vi "Countdown (SubVI).vi"(9 "s":bool) -> (0 "x/y":dbl format="%<%M:%S>t")   [LabVIEW 2020]
panel:
  out "8bit integer 2":i8 format="%08b"
  out "-1, 0, 1":dbl
  out "8bit integer":i8 format="%08b"
  in  "stop":bool
  # "T"
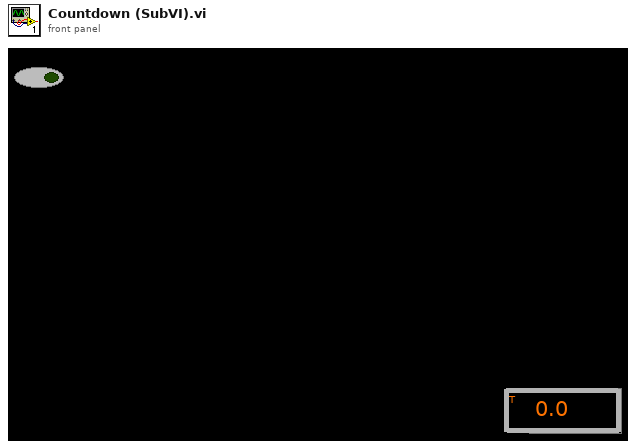
[diagram p1: front panel]
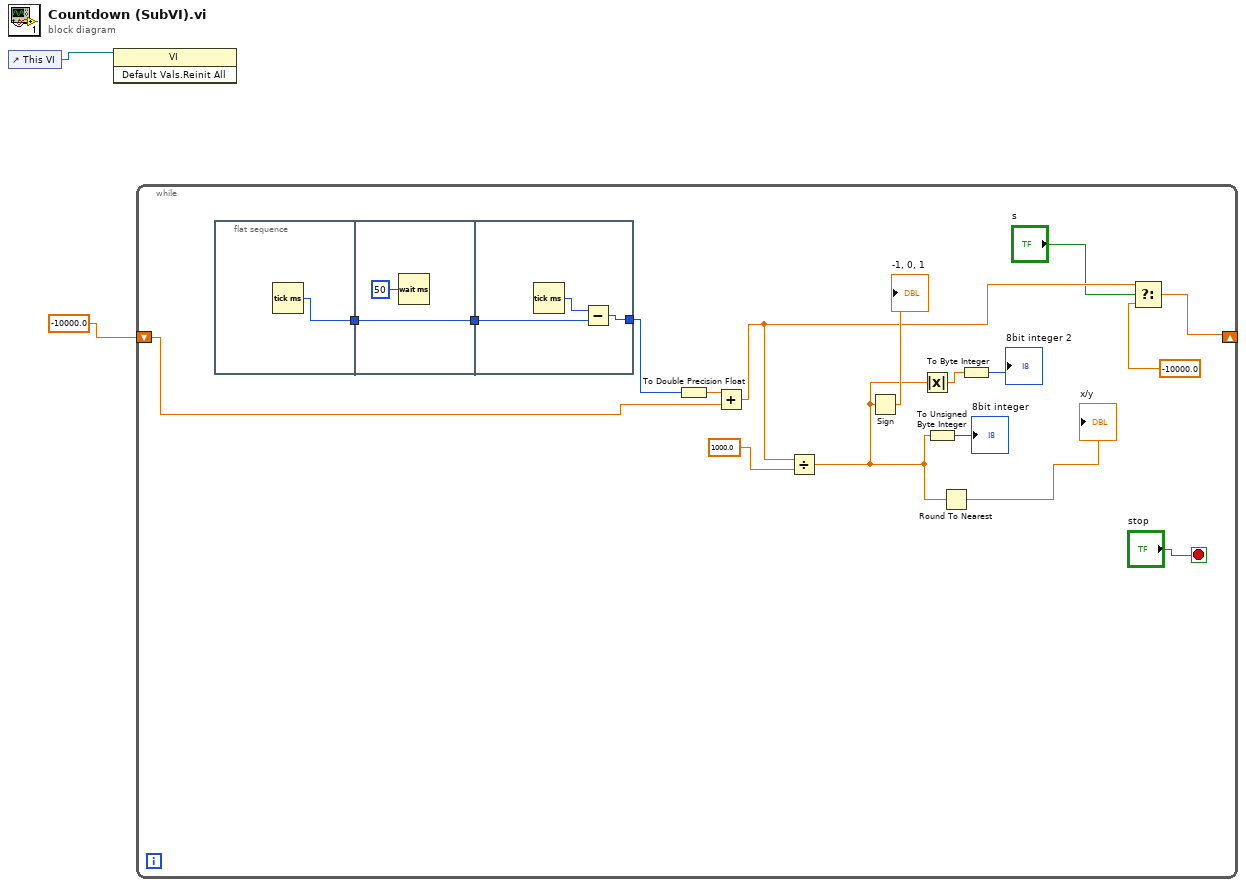
[diagram p0: block diagram]
diagram:
  n1 = control-ref of="This VI"() -> (w2:refnum<vi>)
  n2 = invoke class="VI" method="Default Vals.Reinit All"(reference=w2) -> ()  [unwired: 2 in, 3 out]
  n3 = while {
    shift-right: [w7] -> _
    shift-left: -10000.0 -> [w18]
    stop <- "stop" stop-if-true
    n4 = flat-sequence {
      tunnel: [w20] -> w16
      tunnel: w16 -> [w22]
      tunnel: [w22] -> w15
      tunnel: w15 -> [w24]
      tunnel: [w23] -> w14
      frame #0 {
        n5 = Tick Count (ms)() -> (millisecond timer value=w20:u32)
      }
      frame #1 {
        n6 = Wait (ms)(milliseconds to wait=u32 50) -> ()  [unwired: 1 out]
      }
      frame #2 {
        n7 = Tick Count (ms)() -> (millisecond timer value=w25:u32)
        n8 = Subtract(x=w25, y=w24) -> (x-y=w23:u32)
      }
    }
    n9 = To Double Precision Float(number=w14) -> (double precision float=w13:dbl)
    n10 = Add(x=w13, y=w18) -> (x+y=w8:dbl)
    n11 = Divide(x=w8, y=1000.0) -> (x/y=w4:dbl)
    n12 = Sign(1:w4) -> (0:→"-1, 0, 1":dbl)
    n13 = Absolute Value(x=w4) -> (abs(x)=w10:dbl)
    n14 = To Unsigned Byte Integer(number=w4) -> (unsigned 8bit integer=→"8bit integer":u8)
    n15 = Round To Nearest(number=w4) -> (nearest integer value=→"x/y":dbl)
    n16 = To Byte Integer(number=w10) -> (8bit integer=→"8bit integer 2":i8)
    n17 = Select(t=w8, s="s", f=-10000.0) -> (s? t:f=w7:dbl)
  }
